vi "PNA_GET_TRACE.vi"(0 "VISA resource name":refnum<visa-resource-name>="TCPIP0::K-Instr0000.local::hislip0::INSTR", 1 "Trace File Path":path, 11 "error in (no error)":errorcluster, 12 "Channel (1)":i32=2, 13 "Trace":i32=2) -> (4 "VISA resource name out":refnum<visa-resource-name>="TCPIP0::K-Instr0000.local::hislip0::INSTR", 15 "error out":errorcluster)   [LabVIEW 2018]
uses:
  <vilib>/Utility/file.llb/Write Delimited Spreadsheet (string).vi
  <vilib>/Utility/file.llb/Write Delimited Spreadsheet (DBL).vi
  lib functions/Agilent ENA Series.lvlib
panel:
  out "Trace":dbl[][](array[numeric])=[[10.0, 10.1, 10.2, 10.3, 10.4, 10.5, 10.6, 10.7, 10.8, 10.9, 11.0, 11.1, 11.2, 11.3, 11.4, 11.5, 11.6, 11.7, 11.8, 11.9, 12.0, 12.1, 12.2, 12.3, 12.4, 12.5, 12.6, 12.7, 12.8, 12.9, 13.0, 13.1, 13.2, 13.3, 13.4, 13.5, 13.6, 13.7, 13.8, 13.9, 14.0, 14.1, 14.2, 14.3, 14.4, 14.5, 14.6, 14.7, 14.8, 14.9, 15.0, 15.1, 15.2, 15.3, 15.4, 15.5, 15.6, 15.7, 15.8, 15.9, 16.0, 16.1, 16.2, 16.3, 16.4, 16.5, 16.6, 16.7, 16.8, 16.9, 17.0, 17.1, 17.2, 17.3, 17.4, 17.5, 17.6, 17.7, 17.8, 17.9, 18.0, 18.1, 18.2, 18.3, 18.4, 18.5, 18.6, 18.7, 18.8, 18.9, 19.0, 19.1, 19.2, 19.3, 19.4, 19.5, 19.6, 19.7, 19.8, 19.9, 20.0, 20.1, 20.2, 20.3, 20.4, 20.5, 20.6, 20.7, 20.8, 20.9, 21.0, 21.1, 21.2, 21.3, 21.4, 21.5, 21.6, 21.7, 21.8, 21.9, 22.0, 22.1, 22.2, 22.3, 22.4, 22.5, 22.6, 22.7, 22.8, 22.9, 23.0, 23.1, 23.2, 23.3, 23.4, 23.5, 23.6, 23.7, 23.8, 23.9, 24.0, 24.1, 24.2, 24.3, 24.4, 24.5, 24.6, 24.7, 24.8, 24.9, 25.0, 25.1, 25.2, 25.3, 25.4, 25.5, 25.6, 25.7, 25.8, 25.9, 26.0, 26.1, 26.2, 26.3, 26.4, 26.5, 26.6, 26.7, 26.8, 26.9, 27.0, 27.1, 27.2, 27.3, 27.4, 27.5, 27.6, 27.7, 27.8, 27.9, 28.0, 28.1, 28.2, 28.3, 28.4, 28.5, 28.6, 28.7, 28.8, 28.9, 29.0, 29.1, 29.2, 29.3, 29.4, 29.5, 29.6, 29.7, 29.8, 29.9, 30.0, 30.1, 30.2, 30.3, 30.4, 30.5, 30.6, 30.7, 30.8, 30.9, 31.0, 31.1, 31.2, 31.3, 31.4, 31.5, 31.6, 31.7, 31.8, 31.9, 32.0, 32.1, 32.2, 32.3, 32.4, 32.5, 32.6, 32.7, 32.8, 32.9, 33.0, 33.1, 33.2, 33.3, 33.4, 33.5, 33.6, 33.7, 33.8, 33.9, 34.0, 34.1, 34.2, 34.3, 34.4, 34.5, 34.6, 34.7, 34.8, 34.9, 35.0, 35.1, 35.2, 35.3, 35.4, 35.5, 35.6, 35.7, 35.8, 35.9, 36.0, 36.1, 36.2, 36.3, 36.4, 36.5, 36.6, 36.7, 36.8, 36.9, 37.0, 37.1, 37.2, 37.3, 37.4, 37.5, 37.6, 37.7, 37.8, 37.9, 38.0, 38.1, 38.2, 38.3, 38.4, 38.5, 38.6, 38.7, 38.8, 38.9, 39.0, 39.1, 39.2, 39.3, 39.4, 39.5, 39.6, 39.7, 39.8, 39.9, 40.0], [-83.75083620343261, -80.72327748123962, -82.02324332268196, -84.68478463283594, -84.15081582655829, -82.5109050366294, -83.63468799788856, -84.6746841995481, -82.36709093602624, -85.28832181781615, -85.97792566528115, -85.29299978675262, -87.25682565458754, -84.2653339756456, -83.22005551141687, -82.34890473787372, -83.25033135737927, -80.96285744101685, -81.14100280010587, -82.7646178861791, -81.79356971250161, -83.37128341668566, -83.20002234609646, -83.09287991871132, -84.2958820179426, -85.78652538726033, -81.39349365381207, -82.19849650445374, -82.26350335743076, -84.31929265179627, -78.30393256357249, -72.51944567195325, -66.51005470163506, -61.859121459218294, -58.07293722888295, -55.28115134560778, -52.778051419413565, -50.33697038412026, -47.79911625891634, -45.756727755421245, -44.138940789312045, -42.147350286738586, -40.4545767956084, -37.60264639256018, -34.863644622442926, -32.40754634793201, -30.846844320850252, -29.71413795154813, -29.47771804614154, -28.94498875687232, -29.093599096562937, -28.62346169363585, -28.2277604534099, -27.932523830432178, -27.5954171999582, -27.249426919963714, -27.513839070982232, -28.31739796256226, -28.621790419592568, -29.172537834278877, -28.571354093695412, -28.108757819444246, -27.158002680191046, -26.492910051023184, -25.847587907608368, -25.346830953327327, -24.679821567981868, -24.64862200127188, -23.900966826318037, -23.261831716034663, -23.40553257114662, -23.531283755440207, -24.0350777448283, -24.472790437350078, -24.895270751380124, -24.788725841612195, -24.57822475065739, -24.26843476384985, -24.276743956960733, -23.972386057009054, -24.44528963925082, -23.995836935866343, -23.290853423514758, -22.403406161428666, -21.49360652751955, -20.803487087502887, -19.77764942662872, -19.454663265301917, -19.206914802011745, -19.486660318844308, -19.49159060421709, -19.069847350144503, -19.270551817103257, -19.343277771711705, -19.349938786747764, -19.362166636504345, -19.17761000125524, -19.131927500735678, -19.766136886130056, -20.143235979589242, -21.343679051741734, -22.12059615332894, -22.98094178984823, -23.487121849157045, -23.396804570111573, -22.89972361504958, -22.51243997923239, -22.597597570254045, -23.163438813935326, -23.273821587922075, -23.333858978952925, -22.78940537861482, -22.285165249522066, -21.74866109545379, -21.662902873388923, -21.228739784001274, -20.835401770909403, -20.612413124528256, -20.43204711197547, -20.25283622988635, -20.22813368040285, -20.159633396583683, -20.426315991368874, -21.236215785122226, -22.171114413483583, -22.639981516991547, -22.801525794065412, -22.846560729199798, -22.409407941719618, -22.71573710327261, -22.775594005714037, -22.861831340483082, -23.386709911336382, -23.56564287639189, -23.965958519444023, -23.97253123998105, -24.621686761082962, -24.77499094197257, -25.57055748239323, -25.243509020986377, -24.39111757991789, -23.725827886141314, -23.32477562906115, -22.90761588879271, -22.78862828485685, -22.969526827358123, -23.417196033655692, -24.58570559672455, -25.53828398293065, -27.033519521552094, -27.389581554722024, -27.51226831761292, -27.84528470936511, -28.07216191068459, -28.307884494251194, -28.01840054524826, -27.67026757023999, -27.730283736947175, -28.412863839600284, -29.216708623137485, -30.24562476419829, -30.719416693555708, -31.52674084793995, -32.15436814899731, -32.74580270060876, -33.838180896394825, -34.84606069652151, -35.65608662594705, -35.933505033524575, -36.05972366701665, -36.6067555131147, -37.13137091550151, -37.85439730857892, -38.49694550249322, -39.514382373124086, -40.387685538157214, -42.205117703388105, -43.63415412505301, -46.073947128023924, -47.847207948977186, -49.2772882383644, -51.1143885657503, -52.15656726685278, -53.16356100877658, -54.32452528928942, -57.003022945298284, -59.039672486813444, -59.6457552308895, -60.609321272066325, -62.219451238766936, -62.81956189064253, -63.221465471472925, -64.28666273575524, -64.75488393602996, -66.25600812477286, -66.20366229066019, -68.01892747046138, -68.7596834102592, -68.92966247944996, -69.6800496434035, -70.31058099368654, -70.5536792126986, -72.94189477835451, -73.19909726739562, -75.70325574440575, -75.06756579341369, -77.42811515237581, -78.55199431716473, -75.83697092286283, -73.15076499173499, -74.1961114823993, -75.7723358459186, -77.72837359560401, -74.66913298289643, -77.64420945675481, -77.1212009860575, -76.36359264683756, -75.99500432777545, -75.25512424360339, -73.72148632588197, -78.54116695080447, -76.77572032388858, -75.296651879736, -75.48521020457994, -79.41145213186604, -78.03306797267167, -75.22719128519307, -78.14946891257826, -78.74545703710812, -78.77269536752947, -75.38349164954946, -78.01287135135381, -77.37237127832346, -77.82968576100625, -76.46168775885297, -80.19107498122729, -76.21226276335513, -75.90893568121456, -79.81818238927931, -77.654168327867, -76.93735486891873, -77.57347881476531, -77.77999342516426, -79.02902291590766, -76.66708411930708, -79.11173596490245, -77.89903388085708, -76.57165275372428, -79.60832930097052, -80.58340492426962, -76.53384208369769, -78.68311795428556, -79.69356170429985, -75.9752886147058, -75.06219068869784, -76.67572249942727, -78.05353087745002, -79.95322073655701, -77.32648135693363, -79.88067879728897, -76.89910708021517, -74.57522251006927, -77.10036326519234, -79.12995035706687, -77.77931703816165, -79.74944021049738, -76.25887691998273, -80.24120008344154, -79.2935032328805, -76.43384592424879, -74.86115343236254, -77.5212038988716, -77.09598312025324, -78.29474962287757, -77.41354568319679, -73.99234155086648, -76.12252466369699, -77.28532456471814, -74.85781043175979, -77.07650286927388, -76.01909501620598, -75.8983709167753, -77.01598459062106, -76.3354843832578, -74.32941288304973, -75.57082396818905, -75.96689969103677, -73.65676418532632, -75.64364203841771, -77.3167146646185, -76.19513975721236, -75.1542501271011, -73.70872403359266, -76.77791108428599, -72.32512252343147, -73.92695093232548, -73.54650216868721, -78.12864653821575, -76.8442533864186, -73.79272121652009, -73.93727298529633]]
  in  "Correction (0: Data)":u16(ring)=1 items=["Formatted", "Corrected"]
  in  "Source (0: Data)":u16(ring) items=["Data", "Memory"]
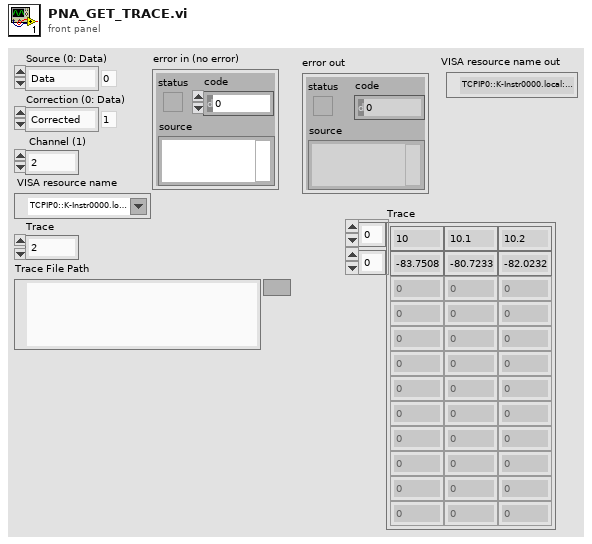
[diagram p1: front panel]
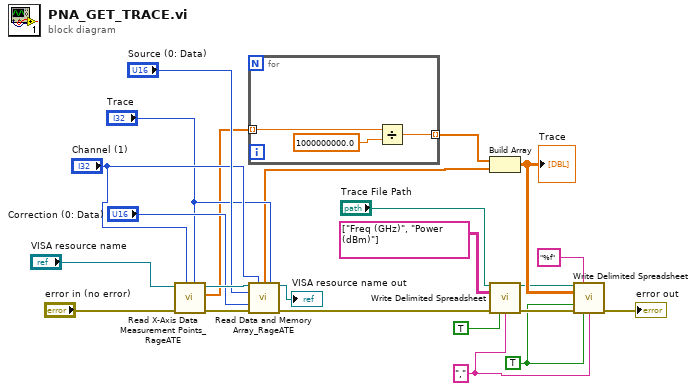
[diagram p0: block diagram]
diagram:
  w4 = "," ("delimiter (\\t)")
  w5 = TRUE ("transpose? (no:F)")
  n1 = call "Read X-Axis Data Measurement Points_RageATE.vi"("Trace"="Trace", "Channel (1)"="Channel (1)", "error in (no error)"="error in (no error)", "VISA resource name"="VISA resource name") -> ("error out"=w22:errorcluster, "X-Axis Data Measurement Points"=w3:dbl[], "VISA resource name out"=w23:refnum<visa-resource-name>)  [unwired: 5 in]
  n2 = for {
    tunnel: w3 -> [w26] mode=indexing
    tunnel: [w25] -> w2 mode=indexing
    n3 = Divide(x=w26, y=1000000000.0) -> (x/y=w25:dbl)
  }
  n4 = call "Read Data and Memory Array_RageATE.vi"("VISA resource name"=w23, "Channel (1)"="Channel (1)", "Trace"="Trace", "Source (0: Data)"="Source (0: Data)", "Correction (0: Data)"="Correction (0: Data)", "error in (no error)"=w22) -> ("dB"=w12:dbl[], "VISA resource name out"=→"VISA resource name out":refnum<visa-resource-name>, "error out"=w9:errorcluster)  [unwired: 5 in, 2 out]
  n5 = Build Array(w2, w12) -> (w14:dbl[][])
  "Trace" <- w14
  n6 = call-poly <vilib>:"Write Delimited Spreadsheet.vi"("file path (dialog if empty)"="Trace File Path", "2D data"=string[][] [["Freq (GHz)"], ["Power (dBm)"]], "error in (no error)"=w9, "transpose? (no:F)"=TRUE, "delimiter (\\t)"=w4) -> ("new file path (Not A Path if cancelled)"=w11:path, "error out"=w8:errorcluster)  [unwired: 9 in]
  n7 = call-poly <vilib>:"Write Delimited Spreadsheet.vi"("file path (dialog if empty)"=w11, "format (%.3f)"="%f", "2D data"=w14, "append to file? (new file:F)"=w5, "error in (no error)"=w8, "transpose? (no:F)"=w5, "delimiter (\\t)"=w4) -> ("error out"=→"error out":errorcluster)  [unwired: 7 in, 1 out]
